vi "File to Configuration.vi"(8 "error in (no error)":errorcluster, 11 "configuration path in":path) -> (0 "error out":errorcluster, 2 "configuration":T1, 3 "configuration path out":path)   [LabVIEW 2017, in "DSF Core.lvlib" / "Configuration Session.lvclass"]
uses:
  Configuration Session.lvclass
  Internal DSF Channel Info.ctl
  Internal DSF Channel with ID.ctl
  Internal DSF Transfer Info.ctl
  Internal DSF Transfer with ID.ctl
  Typedefs/DSF Timing Info.ctl
  DSF Core.lvlib
  Internal DSF Group Info.ctl
  Internal DSF Group with ID.ctl
  Typedefs/DSF Settings Info.ctl
  Typedefs/DSF Engine Plugin Thread Configuration.ctl
  Internal DSF Plugin Info.ctl
  Internal DSF Plugin with ID.ctl
  Typedefs/DSF Version Info.ctl
  Internal DSF Settings Info.ctl
  Internal DSF Settings with ID.ctl
  Typedefs/DSF Engine Framework Configuration.ctl
  Internal DSF Configuration.ctl
  Typedefs/DSF Direction.ctl
  Typedefs/DSF Byte Order.ctl
  Typedefs/DSF Data Type.ctl
  Typedefs/DSF Engine Channel Configuration.ctl
  Typedefs/DSF Engine Transfer Configuration.ctl
  Typedefs/DSF Timeout Behavior.ctl
  Typedefs/DSF Engine Transfer Group Configuration.ctl
  Typedefs/DSF Engine Plugin Configuration.ctl
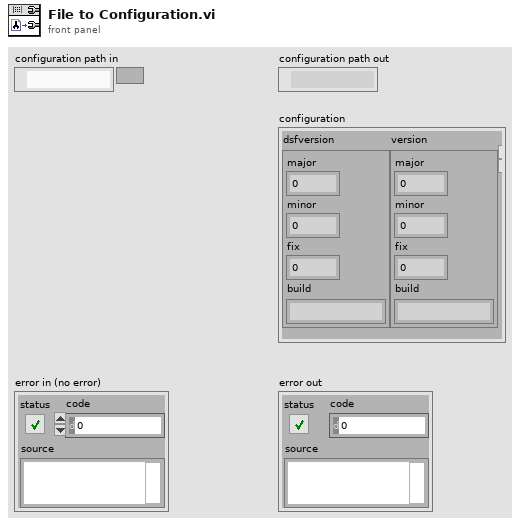
[diagram p1: front panel]
types:
  T1 = typedef "DSF Core.lvlib/Configuration Session.lvclass/Internal DSF Configuration.ctl" = cluster{"dsfversion":T2, "version":T2, "plugins":T3[], "groups":T8[], "transfers":T10[], "channels":T12[], "settings":T14[], "framework configuration":T16}
  T2 = typedef "DSF Core.lvlib/DSF Version Info.ctl" = cluster{"major":i32, "minor":i32, "fix":i32, "build":string}
  T3 = typedef "DSF Core.lvlib/Configuration Session.lvclass/Internal DSF Plugin with ID.ctl" = cluster{"id":string, "values":T4}
  T4 = typedef "DSF Core.lvlib/Configuration Session.lvclass/Internal DSF Plugin Info.ctl" = cluster{"components":string[], "timing":T5, "group ids":string[], "settings id":string, "threads":T6[]}
  T5 = typedef "DSF Core.lvlib/DSF Timing Info.ctl" = cluster{"priority":u64, "decimation":u64, "offset":u64}
  T6 = typedef "DSF Core.lvlib/DSF Engine Plugin Thread Configuration.ctl" = cluster{"processor":i32, "priority offset":i16, "settings":T7}
  T7 = typedef "DSF Core.lvlib/DSF Settings Info.ctl" = cluster{"component":string, "name":string, "values":cluster{"key":string, "value":string}[]}[]
  T8 = typedef "DSF Core.lvlib/Configuration Session.lvclass/Internal DSF Group with ID.ctl" = cluster{"id":string, "values":T9}
  T9 = typedef "DSF Core.lvlib/Configuration Session.lvclass/Internal DSF Group Info.ctl" = cluster{"direction":i32, "timing":T5, "transfer ids":string[], "settings id":string, "thread":i32, "timeout behavior":u8}
  T10 = typedef "DSF Core.lvlib/Configuration Session.lvclass/Internal DSF Transfer with ID.ctl" = cluster{"id":string, "values":T11}
  T11 = typedef "DSF Core.lvlib/Configuration Session.lvclass/Internal DSF Transfer Info.ctl" = cluster{"byte order":i32, "channel ids":string[], "settings id":string}
  T12 = typedef "DSF Core.lvlib/Configuration Session.lvclass/Internal DSF Channel with ID.ctl" = cluster{"id":string, "values":T13}
  T13 = typedef "DSF Core.lvlib/Configuration Session.lvclass/Internal DSF Channel Info.ctl" = cluster{"string buffer offset":u64, "string data type":i32, "engine data type":i32, "settings id":string, "units":string}
  T14 = typedef "DSF Core.lvlib/Configuration Session.lvclass/Internal DSF Settings with ID.ctl" = cluster{"id":string, "values":T15}
  T15 = typedef "DSF Core.lvlib/Configuration Session.lvclass/Internal DSF Settings Info.ctl" = cluster{"key":string, "value":string}[]
  T16 = typedef "DSF Core.lvlib/DSF Engine Framework Configuration.ctl" = cluster{"plugins":T17[]}
  T17 = typedef "DSF Core.lvlib/DSF Engine Plugin Configuration.ctl" = cluster{"name":string, "components":string[], "cycle timing":T5, "threads":T6[], "transfer groups":T18[], "settings":T7}
  T18 = typedef "DSF Core.lvlib/DSF Engine Transfer Group Configuration.ctl" = cluster{"name":string, "direction":T19, "cycle timing":T5, "thread index":u8, "settings":T7, "transfers":T20[], "timeout behavior":T24, "convert buffers":bool}
  T19 = typedef "DSF Core.lvlib/DSF Direction.ctl" = enum8{"Tx", "Rx"}
  T20 = typedef "DSF Core.lvlib/DSF Engine Transfer Configuration.ctl" = cluster{"name":string, "string byte order":T21, "settings":T7, "channels":T22[]}
  T21 = typedef "DSF Core.lvlib/DSF Byte Order.ctl" = enum8{"big-endian", "little-endian"}
  T22 = typedef "DSF Core.lvlib/DSF Engine Channel Configuration.ctl" = cluster{"string offset":u64, "name":string, "units":string, "engine data type":T23, "string data type":T23, "settings":T7}
  T23 = typedef "DSF Core.lvlib/DSF Data Type.ctl" = enum8{"Bool", "SGL", "DBL", "I8", "I16", "I32", "I64", "U8", "U16", "U32", "U64"}
  T24 = typedef "DSF Core.lvlib/DSF Timeout Behavior.ctl" = enum8{"Increment Late Count", "Throw Error"}
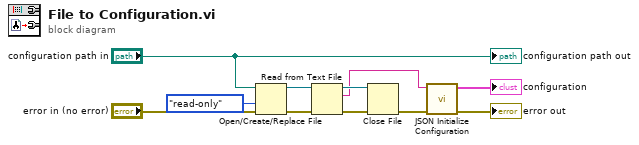
[diagram p0: block diagram]
diagram:
  n1 = Open/Create/Replace File(file path (use dialog)="configuration path in", error in="error in (no error)", access (0:read/write)=enum16{"read/write", "read-only", "write-only"}."read-only") -> (refnum out=w6:refnum<file>, error out=w10:errorcluster)  [unwired: 4 out]
  n2 = Read from Text File(file (use dialog)=w6, error in=w10) -> (refnum out=w5:refnum<file>, text=w3:string, error out=w9:errorcluster)  [unwired: 3 out]
  n3 = Close File(refnum=w5, error in=w9) -> (error out=w4:errorcluster)  [unwired: 1 out]
  n4 = call "JSON Initialize Configuration.vi"("error in (no error)"=w4, "file json"=w3) -> ("error out"=→"error out":errorcluster, "config data"=→"configuration":T1)  [unwired: 8 in]
  "configuration path out" <- "configuration path in"
